vi "Get Ball Header.vi"(1 "Camera Res X":i32, 2 "Ranked Objects":T1(array[cluster]) {"Score" format="%#.1g"}) -> (0 "Angle X":dbl)   [LabVIEW 2013]
doc: "Given a ball's pixel coordinates, calculate a horizontal angle to the center of the ball."
panel:
  in  "Camera FOV X":dbl=67.0
  # "Make sure this is accurate for the camera that is being used."
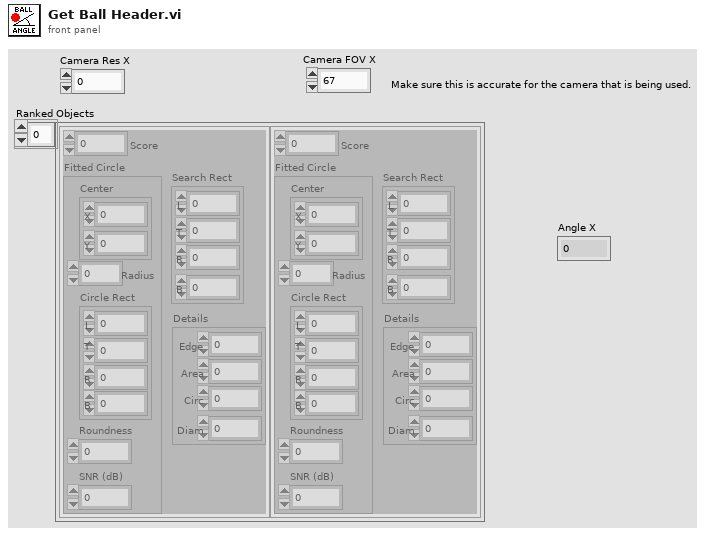
[diagram p1: front panel]
types:
  T1 = cluster{"Score":sgl, "Fitted Circle":cluster{"Center":cluster{"X":sgl, "Y":sgl}, "Radius":dbl, "Circle Rect":cluster{"L":sgl, "T":sgl, "R":sgl, "B":sgl}, "Roundness":dbl, "SNR (dB)":dbl}, "Search Rect":cluster{"L":sgl, "T":sgl, "R":sgl, "B":sgl}, "Details":cluster{"Edge":sgl, "Area":sgl, "Circ":sgl, "Diam":sgl}}[]
  T2 = cluster{"Score":sgl, "Fitted Circle":cluster{"Center":cluster{"X":sgl, "Y":sgl}, "Radius":dbl, "Circle Rect":cluster{"L":sgl, "T":sgl, "R":sgl, "B":sgl}, "Roundness":dbl, "SNR (dB)":dbl}, "Search Rect":cluster{"L":sgl, "T":sgl, "R":sgl, "B":sgl}, "Details":cluster{"Edge":sgl, "Area":sgl, "Circ":sgl, "Diam":sgl}}
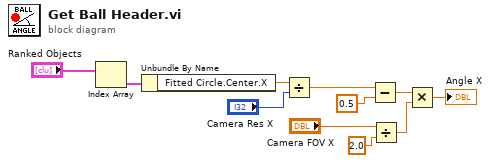
[diagram p0: block diagram]
diagram:
  n1 = Index Array(array="Ranked Objects") -> (element=w6:T2)  [unwired: 1 in]
  n2 = Unbundle By Name(w6) -> ("Fitted Circle.Center.X"=w2:sgl)
  n3 = Divide(x=w2, y="Camera Res X") -> (x/y=w10:sgl)
  n4 = Subtract(x=w10, y=0.5) -> (x-y=w8:dbl)
  n5 = Divide(x="Camera FOV X", y=2.0) -> (x/y=w4:dbl)
  n6 = Multiply(x=w8, y=w4) -> (x*y=→"Angle X":dbl)
